vi "FGV DB Variant.vi"(9 "Data":variant, 10 "name":string, 11 "Opcion":enum16{"Set Data", "Get Data", "Reset Data"}(ring)) -> (1 "found?":bool, 2 "replaced?":bool, 3 "value":variant)   [LabVIEW 2019]
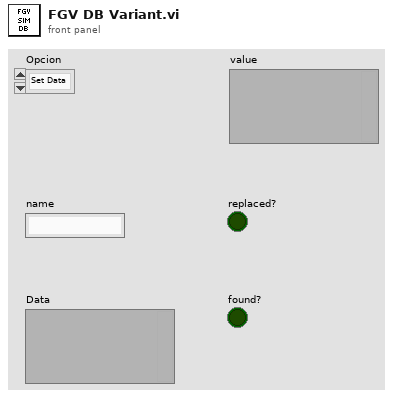
[diagram p1: front panel]
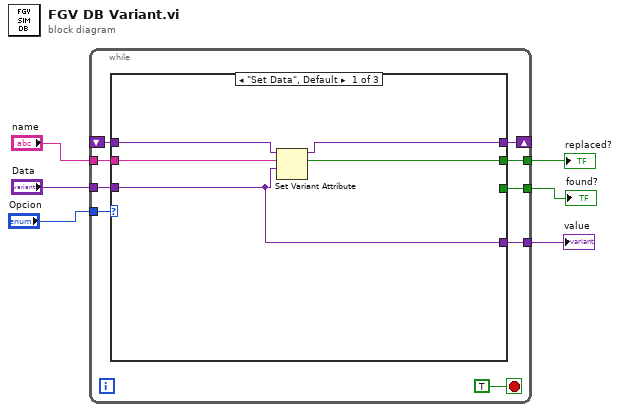
[diagram p0: block diagram]
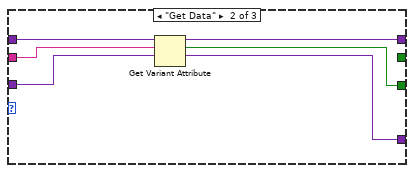
[diagram p2: hidden frame]
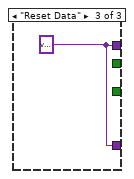
[diagram p3: hidden frame]
diagram:
  n1 = while {
    tunnel: "Opcion" -> [w14]
    shift-right: [w13] -> _
    shift-left: _ -> [w12]
    tunnel: "name" -> [w11]
    tunnel: "Data" -> [w10]
    tunnel: [w9] -> w3
    tunnel: [w8] -> w2
    tunnel: [w7] -> w1
    stop <- TRUE stop-if-true
    n2 = case shown="\"Set Data\", Default" w14 {
      tunnel: [w20 w25 w27] -> w13
      tunnel: w12 -> [w19 w26 _]
      tunnel: w11 -> [w18 w24 _]
      tunnel: w10 -> [w16 w23 _]
      tunnel: [w17 _ _] -> w9
      tunnel: [_ w22 _] -> w8
      tunnel: [w16 w21 w27] -> w7
      frame "Set Data", Default {
        n3 = Set Variant Attribute(Variant=w19, name=w18, value=w16) -> (Variant out=w20:variant, replaced=w17:bool)  [unwired: 1 in, 1 out]
      }
      frame "Get Data" {
        n4 = Get Variant Attribute(Variant=w26, name=w24, default value (empty Variant)=w23) -> (duplicate Variant=w25:variant, found=w22:bool, value=w21:variant)  [unwired: 1 in, 1 out]
      }
      frame "Reset Data" {
        w27 = variant
      }
    }
  }
  "replaced?" <- w3
  "found?" <- w2
  "value" <- w1
